vi "JSON Delta RR Update.vi"(9 "Delta JSON":string, 11 "input":T1={"type"="roboRIO", "device"="", "name"="", "data"={">fpga_button"=FALSE, ">vin_voltage"=0.0, ">vin_current"=0.0, ">6v_voltage"=0.0, ">6v_current"=0.0, ">6v_active"=FALSE, ">6v_faults"=0.0, ">5v_voltage"=0.0, ">5v_current"=0.0, ">5v_active"=FALSE, ">5v_faults"=0.0, ">3v3_voltage"=0.0, ">3v3_current"=0.0, ">3v3_active"=FALSE, ">3v3_faults"=0.0}}) -> (0 "error out":errorcluster, 3 "output":T1={"type"="roboRIO", "device"="", "name"="", "data"={">fpga_button"=FALSE, ">vin_voltage"=0.0, ">vin_current"=0.0, ">6v_voltage"=0.0, ">6v_current"=0.0, ">6v_active"=FALSE, ">6v_faults"=0.0, ">5v_voltage"=0.0, ">5v_current"=0.0, ">5v_active"=FALSE, ">5v_faults"=0.0, ">3v3_voltage"=0.0, ">3v3_current"=0.0, ">3v3_active"=FALSE, ">3v3_faults"=0.0}})   [LabVIEW 2019]
uses:
  RoboRIO data proto.ctl
  RoboRIO proto.ctl
panel:
  out "JSON of original":string
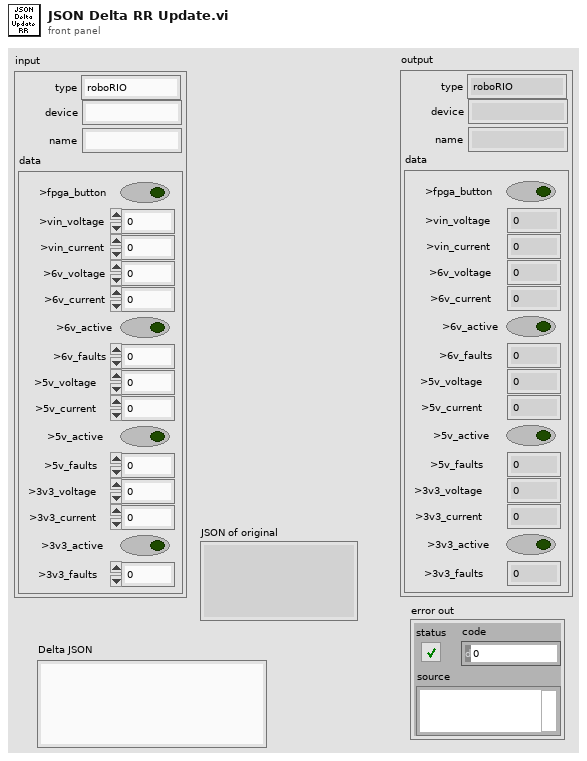
[diagram p1: front panel]
types:
  T1 = typedef "RoboRIO proto.ctl" = cluster{"type":string, "device":string, "name":string, "data":T2}
  T2 = typedef "RoboRIO data proto.ctl" = cluster{">fpga_button":bool, ">vin_voltage":dbl, ">vin_current":dbl, ">6v_voltage":dbl, ">6v_current":dbl, ">6v_active":bool, ">6v_faults":dbl, ">5v_voltage":dbl, ">5v_current":dbl, ">5v_active":bool, ">5v_faults":dbl, ">3v3_voltage":dbl, ">3v3_current":dbl, ">3v3_active":bool, ">3v3_faults":dbl}
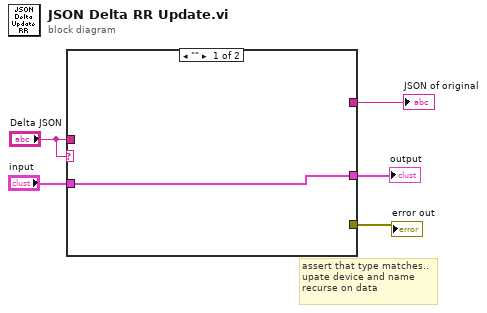
[diagram p0: block diagram]
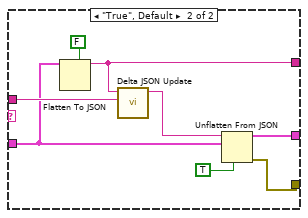
[diagram p2: hidden frame]
diagram:
  # "assert that type matches..\nupate device and name\nrecurse on data"
  n1 = case shown="\"\"" "Delta JSON" {
    tunnel: [_ w13] -> w5
    tunnel: "Delta JSON" -> [_ w11]
    tunnel: [_ w10] -> w4
    tunnel: "input" -> [w6 w8]
    tunnel: [w6 w7] -> w2
    frame "" {
    }
    frame "True", Default {
      n2 = Flatten To JSON(enable LabVIEW extensions? (T)=FALSE, anything=w8) -> (JSON string=w13:string)  [unwired: 1 in, 1 out]
      n3 = call "Delta JSON Update.vi"("Delta JSON"=w11, "JSON string in"=w13) -> ("JSON string out"=w12:string)  [unwired: 9 in]
      n4 = Unflatten From JSON(JSON string=w12, type and defaults=w8, default null elements? (F)=TRUE) -> (value=w7:T1, error out=w10:errorcluster)  [unwired: 4 in]
    }
  }
  "JSON of original" <- w5
  "error out" <- w4
  "output" <- w2
